vi "Convert API String Arguments to Data Variant.vi"(7 "Type":variant, 11 "String":string) -> (1 "error":errorcluster, 3 "Data":variant)   [LabVIEW 2020, in "JKISM++ API String Arguments Support.lvlib"]
uses:
  JKISM++ API String Arguments Support.lvlib
  <vilib>/Utility/Data Type/Type Definitions/Data Type.ctl
  <userlib>/NEVSTOP-Programming-Palette/Numeric/_Instance/String To Number(I64)_nevstop.vi
  <userlib>/_OpenG.lib/string/string.llb/Trim Whitespace__ogtk.vi
  <userlib>/_OpenG.lib/string/string.llb/Trim Whitespace (String)__ogtk.vi
  <vilib>/Utility/Data Type/NI_Data Type.lvlib
  <userlib>/_NEVSTOP/JKI State Machine++/JKI State Machine++.lvlib
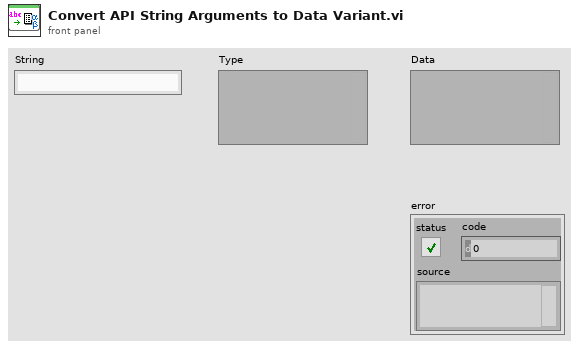
[diagram p1: front panel]
types:
  T1 = typedef "NI_Data Type.lvlib/Data Type.ctl" = enum8{"Invalid Type", "Void", "I8", "I16", "I32", "I64", "U8", "U16", "U32", "U64", "Single Float", "Double Float", "Extended Float", "Single Complex", "Double Complex", "Extended Complex", "Enum U8", "Enum U16", "Enum U32", "Enum U64", "Single Float With Unit", "Double Float With Unit", "Extended Float With Unit", "Single Complex with Unit", "Double Complex with Unit", "Extended Complex with Unit", "Boolean", "String", "Path", "Picture", "Tag", "Array", "Cluster", "Variant", "LV Variant", "Waveform", "Timestamp", "Digital Waveform", "Digital Data", "ExpressData", "Refnum", "External Data", "VI", "Poly VI", "LabVIEW Class Instance", "Fixed Point", "Set Collection", "Map Collection"}
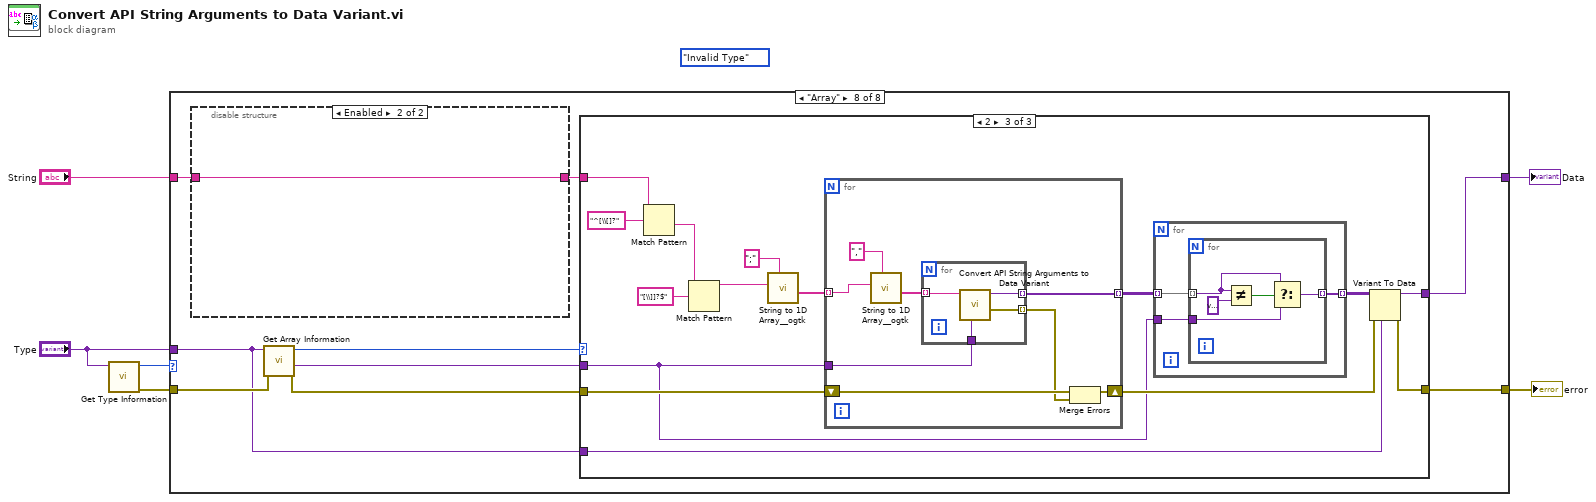
[diagram p0: block diagram]
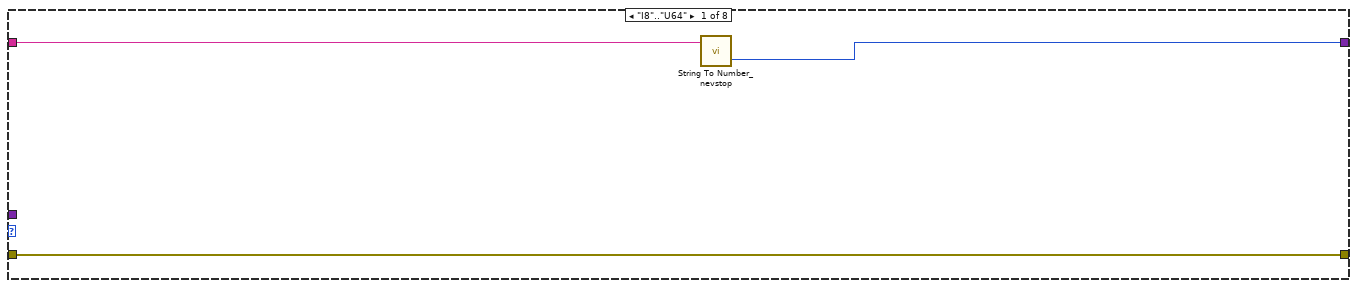
[diagram p2: hidden frame]
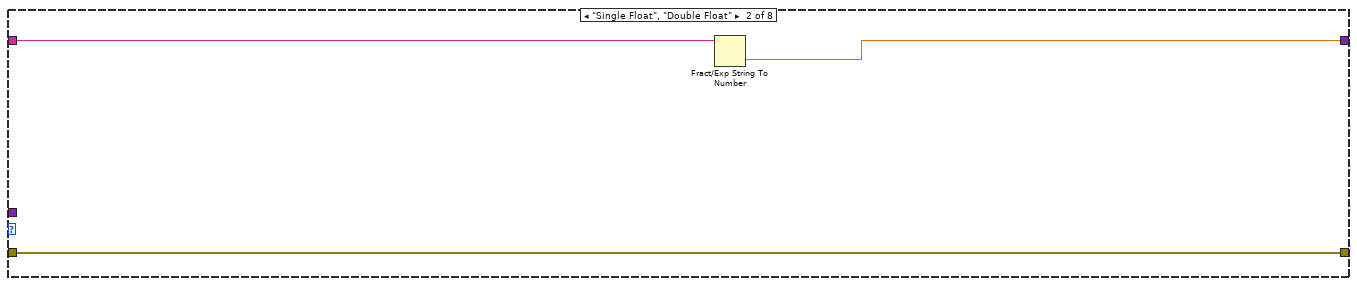
[diagram p3: hidden frame]
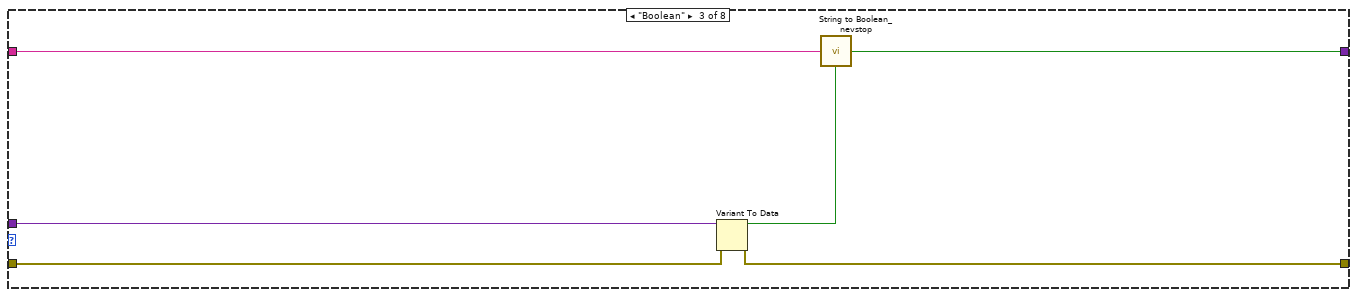
[diagram p4: hidden frame]
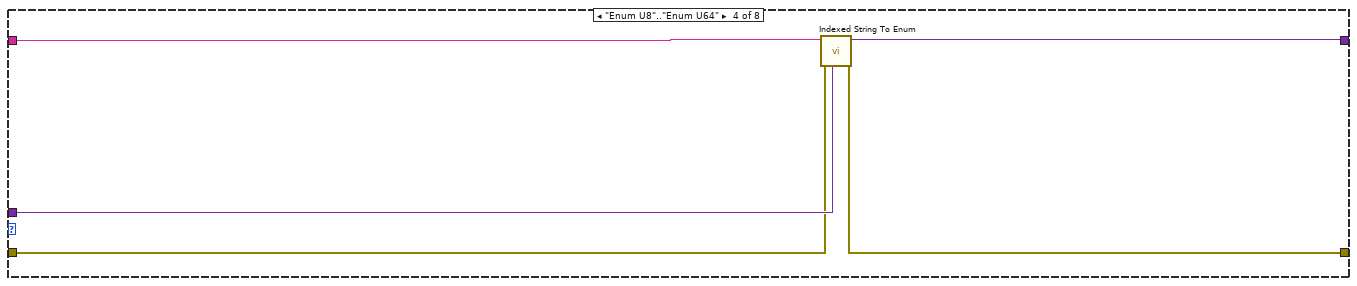
[diagram p5: hidden frame]
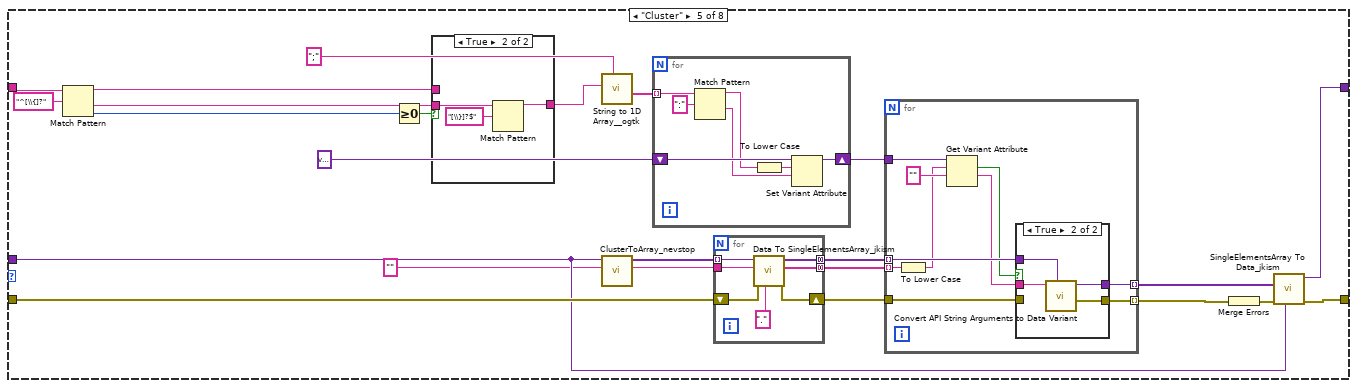
[diagram p6: hidden frame]
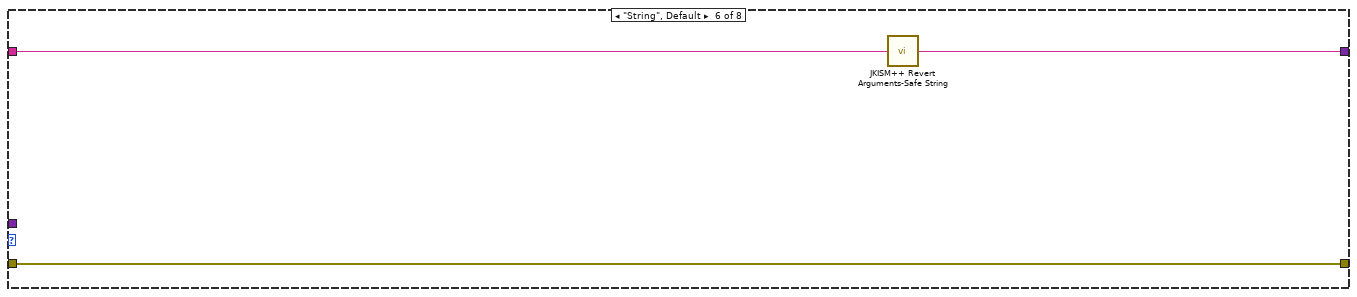
[diagram p9: hidden frame]
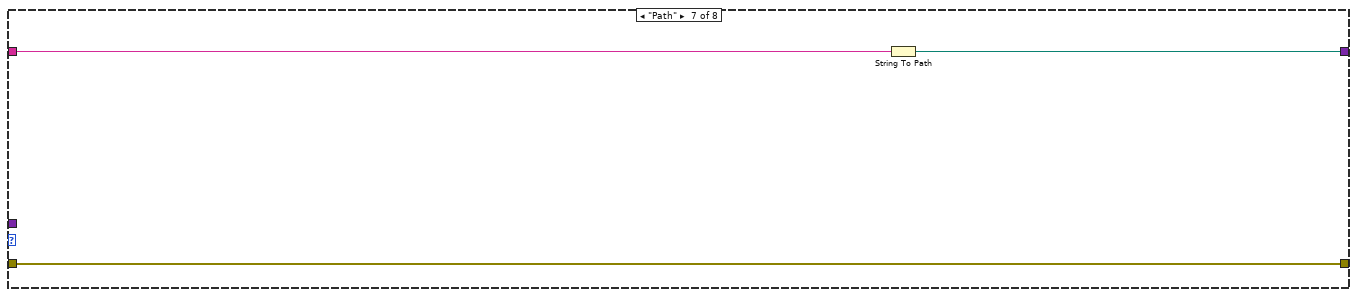
[diagram p10: hidden frame]
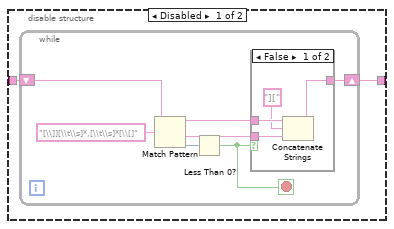
[diagram p11: hidden frame]
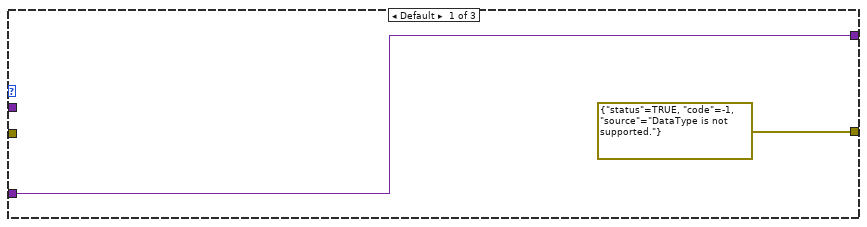
[diagram p13: hidden frame]
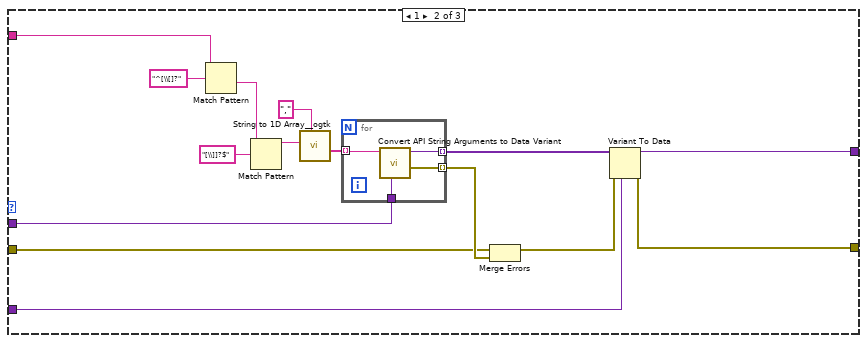
[diagram p14: hidden frame]
diagram:
  (unwired) Data_Type."Invalid Type" ("type")
  n1 = call <vilib>:"Get Type Information.vi"("variant"="Type") -> ("error out"=w5:errorcluster, "type"=w6:T1)  [unwired: 6 in, 3 out]
  n2 = case shown="\"Array\"" w6 {
    tunnel: w5 -> [w7 w12 w14 w21 w45 w83 w86 w95]
    tunnel: [w7 w12 w13 w20 w36 w83 w86 w93] -> w4
    tunnel: [w8 w10 w17 w19 w34 w81 w84 w94] -> w3
    tunnel: "Type" -> [_ _ w16 w22 w33 _ _ w89]
    tunnel: "String" -> [w9 w11 w18 w23 w28 w82 w85 w88]
    frame "I8".."U64" {
      n3 = call-poly <userlib>:"String To Number_nevstop.vi"("String"=w9) -> ("Numeric(I64)"=w8:i64)  [unwired: 4 in]
    }
    frame "Single Float", "Double Float" {
      n4 = Fract/Exp String To Number(string=w11) -> (number=w10:dbl)  [unwired: 3 in, 1 out]
    }
    frame "Boolean" {
      n5 = Variant To Data(error in=w14, Variant=w16) -> (data=w15:bool, error out=w13:errorcluster)  [unwired: 1 in]
      n6 = call <userlib>:"String to Boolean_nevstop.vi"("Default(F)"=w15, "String"=w18) -> ("Boolean"=w17:bool)  [unwired: 2 in]
    }
    frame "Enum U8".."Enum U64" {
      n7 = call <userlib>:"Indexed String To Enum.vi"("Variant"=w22, "error in (no error)"=w21, "String"=w23) -> ("error out"=w20:errorcluster, "Enum"=w19:variant)  [unwired: 7 in]
    }
    frame "Cluster" {
      n8 = Match Pattern(string=w28, regular expression="^[\\{]?") -> (before substring=w24:string, after substring=w30:string, offset past match=w26:i32)  [unwired: 1 in, 1 out]
      n9 = Greater Or Equal To 0?(x=w26) -> (x >= 0?=w25:bool)
      n10 = case shown="True" w25 {
        tunnel: w30 -> [_ w50]
        tunnel: [w47 w48] -> w27
        tunnel: w24 -> [w47 _]
        frame False {
        }
        frame True {
          n11 = Match Pattern(string=w50, regular expression="[\\}]?$") -> (before substring=w48:string)  [unwired: 1 in, 3 out]
        }
      }
      n12 = call <userlib>:"String to 1D Array__ogtk.vi"("delimiter (Tab)"=";", "string"=w27) -> ("Array of Strings"=w44:string[])  [unwired: 9 in]
      n13 = call <userlib>:"ClusterToArray_nevstop.vi"("Cluster"=w33) -> ("Array"=w31:variant[])  [unwired: 10 in]
      n14 = for {
        tunnel: w44 -> [w78] mode=indexing
        shift-right: [w79] -> w42
        shift-left: variant -> [w80]
        n15 = Match Pattern(string=w78, regular expression=":") -> (before substring=w75:string, after substring=w76:string)  [unwired: 1 in, 2 out]
        n16 = To Lower Case(string=w75) -> (all lower case string=w74:string)
        n17 = Set Variant Attribute(Variant=w80, name=w74, value=w76) -> (Variant out=w79:variant)  [unwired: 1 in, 2 out]
      }
      n18 = for {
        tunnel: [w55] -> w41 mode=concatenating
        tunnel: [w53] -> w39 mode=concatenating
        tunnel: "" ("parentUrl") -> [w52]
        tunnel: w31 -> [w51] mode=indexing
        shift-right: [w54] -> w40
        shift-left: w45 -> [w57]
        n19 = call "Data To SingleElementsArray_jkism.vi"("Seperator(/)"=".", "error in (no error)"=w57, "parentUrl"=w52, "Cluster"=w51) -> ("error out"=w54:errorcluster, "Full NameList"=w53:string[], "DataElementArray"=w55:variant[])  [unwired: 5 in]
      }
      n20 = for {
        tunnel: w42 -> [w67]
        tunnel: w41 -> [w64] mode=indexing
        tunnel: w40 -> [w59]
        tunnel: w39 -> [w66] mode=indexing
        tunnel: [w62] -> w37 mode=indexing
        tunnel: [w61] -> w38 mode=indexing
        n21 = To Lower Case(string=w66) -> (all lower case string=w58:string)
        n22 = Get Variant Attribute(Variant=w67, name=w58, default value (empty Variant)="" ("regular expression")) -> (found=w60:bool, value=w63:string)  [unwired: 1 in, 2 out]
        n23 = case shown="True" w60 {
          tunnel: w64 -> [w69 w73]
          tunnel: w63 -> [_ w70]
          tunnel: [w69 w72] -> w62
          tunnel: [w68 w71] -> w61
          tunnel: w59 -> [w68 _]
          frame False {
          }
          frame True {
            n24 = call "Convert API String Arguments to Data Variant.vi"("Type"=w73, "String"=w70) -> ("error"=w71:errorcluster, "Data"=w72:variant)  [unwired: 8 in]
          }
        }
      }
      n25 = Merge Errors(w38) -> (w35:errorcluster)
      n26 = call "SingleElementsArray To Data_jkism.vi"("Pototype"=w33, "error in (no error)"=w35, "DataElementArray"=w37) -> ("error out"=w36:errorcluster, "Cluster"=w34:variant)  [unwired: 7 in]
    }
    frame "String", Default {
      n27 = call <userlib>:"JKISM++ Revert Arguments-Safe String.vi"("Safe Argurment String"=w82) -> ("Origin Argurment String"=w81:string)  [unwired: 8 in]
    }
    frame "Path" {
      n28 = String To Path(string=w85) -> (path=w84:path)
    }
    frame "Array" {
      n29 = disable-structure shown="Enabled" {
        disable-tunnel: w88 -> [w97 w110]
        disable-tunnel: [w96 w110] -> w87
        frame Disabled {
          n30 = while {
            shift-right: [w100] -> w96
            shift-left: w97 -> [w104]
            stop <- w98 stop-if-true
            n31 = Match Pattern(string=w104, regular expression="[\\]][\\t\\s]*,[\\t\\s]*[\\[]") -> (before substring=w102:string, after substring=w101:string, offset past match=w99:i32)  [unwired: 1 in, 1 out]
            n32 = Less Than 0?(x=w99) -> (x < 0?=w98:bool)
            n33 = case shown="False" w98 {
              tunnel: w102 -> [w108 w109]
              tunnel: w101 -> [w107 _]
              tunnel: [w105 w109] -> w100
              frame False {
                n34 = Concatenate Strings(w108, "][" ("string"), w107) -> (w105:string)
              }
              frame True {
              }
            }
          }
        }
        frame Enabled {
        }
      }
      n35 = call <vilib>:"Get Array Information.vi"("error in (no error)"=w95, "variant"=w89) -> ("error out"=w92:errorcluster, "array element data type"=w91:variant, "number of dimensions"=w90:i32)  [unwired: 6 in, 1 out]
      n36 = case shown="2" w90 {
        tunnel: w87 -> [_ w127 w134]
        tunnel: [w112 w119 w146] -> w94
        tunnel: [errorcluster {"status"=TRUE, "code"=-1, "source"="DataType is not supported."} ("error out") w117 w144] -> w93
        tunnel: w92 -> [_ w116 w143]
        tunnel: w91 -> [_ w115 w138]
        tunnel: w89 -> [w112 w113 w141]
        frame Default {
        }
        frame 1 {
          n37 = Match Pattern(string=w127, regular expression="^[\\[]?") -> (after substring=w124:string)  [unwired: 1 in, 3 out]
          n38 = Match Pattern(string=w124, regular expression="[\\]]?$") -> (before substring=w123:string)  [unwired: 1 in, 3 out]
          n39 = call <userlib>:"String to 1D Array__ogtk.vi"("delimiter (Tab)"=",", "string"=w123) -> ("Array of Strings"=w121:string[])  [unwired: 9 in]
          n40 = for {
            tunnel: w121 -> [w128] mode=indexing
            tunnel: [w130] -> w120 mode=indexing
            tunnel: [w129] -> w114 mode=indexing
            tunnel: w115 -> [w131]
            n41 = call "Convert API String Arguments to Data Variant.vi"("Type"=w131, "String"=w128) -> ("error"=w130:errorcluster, "Data"=w129:variant)  [unwired: 8 in]
          }
          n42 = Merge Errors(w116, w120) -> (w118:errorcluster)
          n43 = Variant To Data(error in=w118, type=w113, Variant=w114) -> (data=w119:variant, error out=w117:errorcluster)
        }
        frame 2 {
          n44 = Match Pattern(string=w134, regular expression="^[\\[]?") -> (after substring=w135:string)  [unwired: 1 in, 3 out]
          n45 = Match Pattern(string=w135, regular expression="[\\]]?$") -> (before substring=w133:string)  [unwired: 1 in, 3 out]
          n46 = call <userlib>:"String to 1D Array__ogtk.vi"("delimiter (Tab)"=";", "string"=w133) -> ("Array of Strings"=w132:string[])  [unwired: 9 in]
          n47 = for {
            tunnel: [w152] -> w140 mode=indexing
            tunnel: w138 -> [w151]
            shift-right: [w154] -> w145
            shift-left: w143 -> [w153]
            tunnel: w132 -> [w147] mode=indexing
            n48 = call <userlib>:"String to 1D Array__ogtk.vi"("delimiter (Tab)"=",", "string"=w147) -> ("Array of Strings"=w149:string[])  [unwired: 9 in]
            n49 = for {
              tunnel: w149 -> [w155] mode=indexing
              tunnel: [w157] -> w148 mode=indexing
              tunnel: [w156] -> w152 mode=indexing
              tunnel: w151 -> [w158]
              n50 = call "Convert API String Arguments to Data Variant.vi"("Type"=w158, "String"=w155) -> ("error"=w157:errorcluster, "Data"=w156:variant)  [unwired: 8 in]
            }
            n51 = Merge Errors(w153, w148) -> (w154:errorcluster)
          }
          n52 = for {
            tunnel: w140 -> [w161] mode=indexing
            tunnel: [w160] -> w139 mode=indexing
            tunnel: w138 -> [w159]
            n53 = for {
              tunnel: w161 -> [w163] mode=indexing
              tunnel: [w162] -> w160 mode=indexing
              tunnel: w159 -> [w164]
              n54 = Not Equal?(x=w163, y=variant ("Data")) -> (x != y?=w165:bool)
              n55 = Select(t=w163, s=w165, f=w164) -> (s? t:f=w162:variant)
            }
          }
          n56 = Variant To Data(error in=w145, type=w141, Variant=w139) -> (data=w146:variant, error out=w144:errorcluster)
        }
      }
    }
  }
  "Data" <- w3
  "error" <- w4
